vi "Process.vi"(8 "error in (no error)":errorcluster, 10 "Pound in":refnum<class "Pound.lvclass">, 11 "Qbus in":refnum<class "Qbus.lvclass">) -> (0 "error out":errorcluster)   [LabVIEW 2017, in "CmsDataEventCreator.lvlib"]
uses:
  <vilib>/addons/InsightCM/Devices/Shared/Cms/CmsDataEventCreator/CmsDataEventCreator.lvlib
  <vilib>/addons/Qbus/Qbus.lvclass
  <vilib>/NI/Software Watchdog/Pound/Pound.lvclass
  <vilib>/addons/InsightCM/Devices/Shared/Cms/CmsDataEventCreator/controls/config.ctl
  <vilib>/addons/TraceLogger/TraceLogger.lvlib
  <vilib>/NI/Software Watchdog/Watchdog/Watchdog.lvclass
  <vilib>/addons/InsightCM/Devices/Shared/Common/DataFlow/DataFlow.lvlib
  <vilib>/addons/InsightCM/Devices/Shared/Common/DataAccumulator/DataAccumulator.lvlib
  <vilib>/addons/InsightCM/Devices/Shared/Common/DataEventCreator/DataEventCreator.lvlib
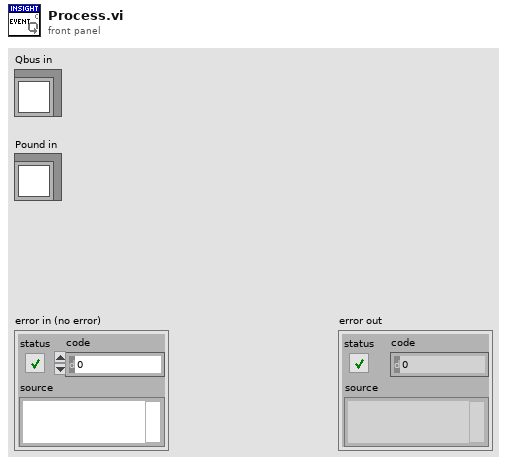
[diagram p1: front panel]
types:
  T1 = typedef "CmsDataEventCreator.lvlib/config.ctl" = cluster{"DeviceName":string, "Groups":string[], "OpenDataEvents":variant, "OpenDataEventConfigs":variant, "AcqParams":variant, "StreamIds":variant, "Registry":variant, "MaxOpenFiles":i32}
  T2 = typedef "DataEventCreator.lvlib/RegisterDataSets.ctl" = cluster{"DataGroup":string, "DataSets":T3[]}
  T3 = typedef "CmsDataEventCreator.lvlib/DataSetRegistry.ctl" = cluster{"ChannelName":string, "DataSetType":T4, "DoNotWriteToDB":bool, "ParentName":string, "CalculateOnServer":bool}
  T4 = typedef "DataEvent.lvlib/DataSetType.ctl" = enum16{"Waveform", "SpeedProfile", "ThermalImage", "EmsaSweep"}
  T5 = typedef "DataEventCreator.lvlib/RegisterTrendPoints.ctl" = cluster{"DataGroup":string, "Trends":T6[]}
  T6 = typedef "DataEventCreator.lvlib/Registry_Trend.ctl" = cluster{"TrendPointId":string, "DataSetName":string, "HighRate":bool, "Always Send":bool}
  T7 = typedef "DataFlow.lvlib/Data.ctl" = cluster{"DataGroup":string, "Waveforms":T8, "Map":T9, "Type":T10}
  T8 = typedef "wfmSGL_DVR.ctl" = refnum<data-value>
  T9 = typedef "PointValueMap.lvlib/PointMap.ctl" = refnum<data-value>
  T10 = typedef "DataFlow.lvlib/Type.ctl" = enum16{"High Rate", "Low Rate", "Burst Mode"}
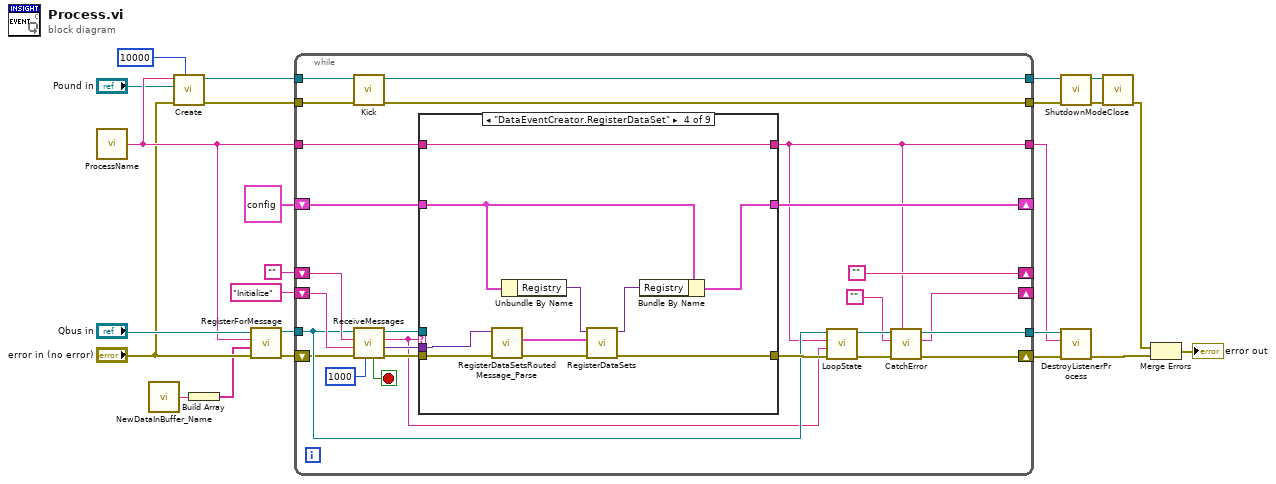
[diagram p0: block diagram]
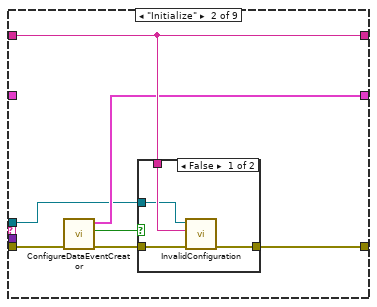
[diagram p3: hidden frame]
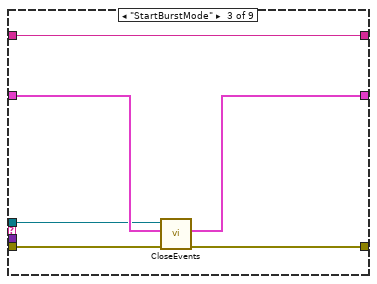
[diagram p5: hidden frame]
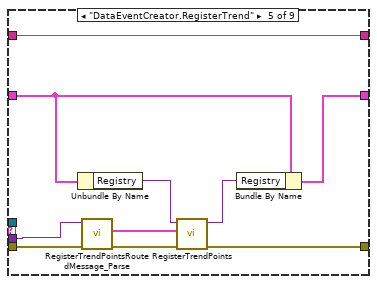
[diagram p6: hidden frame]
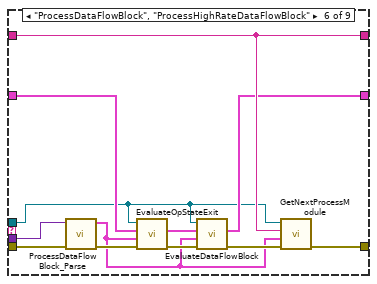
[diagram p7: hidden frame]
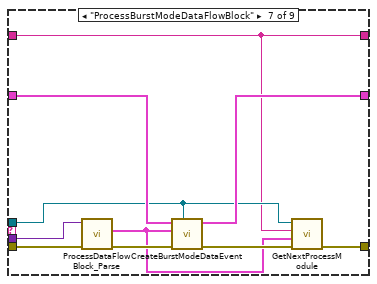
[diagram p8: hidden frame]
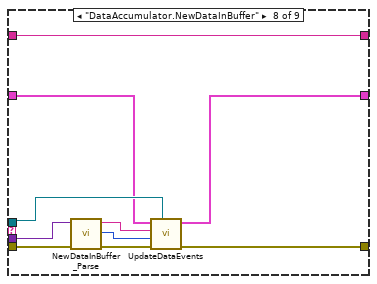
[diagram p9: hidden frame]
diagram:
  n1 = call <vilib>:"ProcessName.vi"() -> ("process name"=w15:string)  [unwired: 5 in]
  n2 = call <vilib>:"NewDataInBuffer_Name.vi"() -> ("MessageName"=w2:string)  [unwired: 5 in]
  n3 = call <vilib>:"Create.vi"("Execution Timeout (ms)"=u32 10000, "error in (no error)"="error in (no error)", "Pound"="Pound in", "Name"=w15) -> ("error out"=w8:errorcluster, "Watchdog"=w14:refnum<data-value>)  [unwired: 6 in]
  n4 = Build Array(w2) -> (w1:string[])
  n5 = call <vilib>:"RegisterForMessage.vi"("error in (no error)"="error in (no error)", "message names"=w1, "process name"=w15, "Qbus in"="Qbus in") -> ("error in (no error)"=w23:errorcluster, "Qbus out"=w22:refnum<class "Qbus.lvclass">)  [unwired: 6 in]
  n6 = while {
    shift-right: [""] -> _
    shift-left: "" -> [w49]
    tunnel: w22 -> [w37]
    tunnel: w15 -> [w27]
    tunnel: [w40] -> w20
    tunnel: [w26] -> w19
    shift-right: [w39] -> _
    shift-left: "Initialize" -> [w44]
    shift-right: [w42] -> _
    shift-left: T1 {"DeviceName"="", "Groups"=[], "OpenDataEvents"=variant(string ""), "OpenDataEventConfigs"=variant, "AcqParams"=variant, "StreamIds"=variant, "Registry"=variant, "MaxOpenFiles"=0} ("config") -> [w43]
    tunnel: w14 -> [w36]
    tunnel: [w35] -> w10
    tunnel: w8 -> [w34]
    tunnel: [w32] -> w7
    shift-right: [w41] -> w21
    shift-left: w23 -> [w33]
    stop <- w50 stop-if-true
    n7 = call <vilib>:"Kick.vi"("error in (no error)"=w34, "Watchdog"=w36) -> ("error out"=w32:errorcluster, "Watchdog"=w35:refnum<data-value>)  [unwired: 8 in]
    n8 = call <vilib>:"ReceiveMessages.vi"("Timeout(1000)"=1000 ("milliseconds to wait"), "error in (no error)"=w33, "priority action"=w44, "default action"=w49, "Qbus in"=w37) -> ("error out"=w48:errorcluster, "message value"=w45:variant, "action"=w31:string, "Qbus out"=w46:refnum<class "Qbus.lvclass">, "exit"=w50:bool)  [unwired: 2 in]
    n9 = case shown="\"DataEventCreator.RegisterDataSet\"" w31 {
      tunnel: w48 -> [w51 w60 w69 w80 w90 w102 w111 w121 w125]
      tunnel: w46 -> [_ w54 w66 _ _ w92 w107 w115 _]
      tunnel: [w51 w58 w70 w76 w85 w101 w106 w118 w125] -> w38
      tunnel: w45 -> [_ _ _ w79 w89 w103 w109 w120 _]
      tunnel: w43 -> [w53 _ w68 w73 w82 w99 w108 w114 w124]
      tunnel: [w53 w55 w67 w72 w86 w94 w112 w113 w124] -> w42
      tunnel: [w52 w56 w71 w81 w91 w100 w105 w122 w123] -> w26
      tunnel: w27 -> [w52 w56 w71 w81 w91 w100 w105 w122 w123]
      frame "", Default {
      }
      frame "Initialize" {
        n10 = call <vilib>:"ConfigureDataEventCreator.vi"("error in (no error)"=w60) -> ("error out"=w59:errorcluster, "valid configuration"=w57:bool, "config"=w55:T1)  [unwired: 8 in]
        n11 = case shown="False" w57 {
          tunnel: w59 -> [w61 w65]
          tunnel: [w64 w65] -> w58
          tunnel: w54 -> [w62 _]
          tunnel: w56 -> [w63 _]
          frame False {
            n12 = call <vilib>:"InvalidConfiguration.vi"("error in (no error)"=w61, "description"=w63, "Qbus in"=w62) -> ("error out"=w64:errorcluster)  [unwired: 7 in, 1 out]
          }
          frame True {
            # "Valid configuration"
          }
        }
      }
      frame "StartBurstMode" {
        n13 = call <vilib>:"CloseEvents.vi"("error in (no error)"=w69, "config in"=w68, "Qbus in"=w66) -> ("error out"=w70:errorcluster, "config out"=w67:T1)  [unwired: 7 in]
      }
      frame "DataEventCreator.RegisterDataSet" {
        n14 = call <vilib>:"RegisterDataSetsRoutedMessage_Parse.vi"("error in (no error)"=w80, "message"=w79) -> ("error out"=w77:errorcluster, "RegisterDataSet"=w78:T2)  [unwired: 8 in]
        n15 = Unbundle By Name(w73) -> ("Registry"=w75:variant)
        n16 = call <vilib>:"RegisterDataSets.vi"("error in (no error)"=w77, "RegisterDataSet"=w78, "registry in"=w75) -> ("error out"=w76:errorcluster, "registry out"=w74:variant)  [unwired: 7 in]
        n17 = Bundle By Name(cluster=w73, "Registry"=w74) -> (w72:T1)
      }
      frame "DataEventCreator.RegisterTrend" {
        n18 = Unbundle By Name(w82) -> ("Registry"=w83:variant)
        n19 = call <vilib>:"RegisterTrendPointsRoutedMessage_Parse.vi"("error in (no error)"=w90, "message"=w89) -> ("error out"=w88:errorcluster, "RegisterTrend"=w84:T5)  [unwired: 8 in]
        n20 = call <vilib>:"RegisterTrendPoints.vi"("error in (no error)"=w88, "register trend"=w84, "registry in"=w83) -> ("error out"=w85:errorcluster, "registry out"=w87:variant)  [unwired: 7 in]
        n21 = Bundle By Name(cluster=w82, "Registry"=w87) -> (w86:T1)
      }
      frame "ProcessDataFlowBlock", "ProcessHighRateDataFlowBlock" {
        n22 = call <vilib>:"ProcessDataFlowBlock_Parse.vi"("error in (no error)"=w102, "body"=w103) -> ("error out"=w96:errorcluster, "data"=w93:T7)  [unwired: 8 in]
        n23 = call <vilib>:"EvaluateOpStateExit.vi"("error in (no error)"=w96, "data flow"=w93, "config"=w99, "Qbus"=w92) -> ("error out"=w97:errorcluster, "config out"=w98:T1)  [unwired: 6 in]
        n24 = call <vilib>:"EvaluateDataFlowBlock.vi"("error in (no error)"=w97, "data"=w93, "config"=w98, "Qbus"=w92) -> ("error out"=w95:errorcluster, "config"=w94:T1)  [unwired: 6 in]
        n25 = call <vilib>:"GetNextProcessModule.vi"("error in (no error)"=w95, "data"=w93, "source"=w100, "Qbus in"=w92) -> ("error out"=w101:errorcluster)  [unwired: 6 in, 1 out]
      }
      frame "ProcessBurstModeDataFlowBlock" {
        n26 = call <vilib>:"ProcessDataFlowBlock_Parse.vi"("error in (no error)"=w111, "body"=w109) -> ("error out"=w110:errorcluster, "data"=w104:T7)  [unwired: 8 in]
        n27 = call <vilib>:"CreateBurstModeDataEvent.vi"("Qbus in"=w107, "error in (no error)"=w110, "data"=w104, "config"=w108) -> ("error out"=w106:errorcluster, "config out"=w112:T1)  [unwired: 6 in]
        n28 = call <vilib>:"GetNextProcessModule.vi"("error in (no error)"=w106, "data"=w104, "source"=w105, "Qbus in"=w107) -> ()  [unwired: 6 in, 2 out]
      }
      frame "DataAccumulator.NewDataInBuffer" {
        n29 = call <vilib>:"NewDataInBuffer_Parse.vi"("error in (no error)"=w121, "Message"=w120) -> ("error out"=w119:errorcluster, "buffer location"=w116:u32, "data group"=w117:string)  [unwired: 7 in]
        n30 = call <vilib>:"UpdateDataEvents.vi"("Qbus"=w115, "error in (no error)"=w119, "buffer location"=w116, "data group"=w117, "config"=w114) -> ("error out"=w118:errorcluster, "config"=w113:T1)  [unwired: 5 in]
      }
      frame "Exit" {
      }
    }
    n31 = call <vilib>:"LoopState.vi"("error in (no error)"=w38, "loop action"=w31, "process name"=w26, "Qbus in"=w37) -> ("error out"=w29:errorcluster, "Qbus out"=w28:refnum<class "Qbus.lvclass">)  [unwired: 6 in]
    n32 = call <vilib>:"CatchError.vi"("source"=w26, "error in (no error)"=w29, "next action in"="", "Qbus in"=w28) -> ("error out"=w41:errorcluster, "next action out"=w39:string, "Qbus out"=w40:refnum<class "Qbus.lvclass">)  [unwired: 5 in]
  }
  n33 = call <vilib>:"ShutdownMode.vi"("error in (no error)"=w7, "Watchdog"=w10) -> ("error out"=w9:errorcluster, "Watchdog"=w11:refnum<data-value>)  [unwired: 8 in]
  n34 = call <vilib>:"DestroyListenerProcess.vi"("error in (no error)"=w21, "process name"=w19, "Qbus in"=w20) -> ("error in (no error)"=w6:errorcluster)  [unwired: 7 in, 1 out]
  n35 = call <vilib>:"Close.vi"("error in (no error)"=w9, "Watchdog"=w11) -> ("error out"=w5:errorcluster)  [unwired: 9 in]
  n36 = Merge Errors(w5, w6) -> (→"error out":errorcluster)
